vi "Data Power Output.vi"(8 "error in (no error)":errorcluster, 11 "PM-EMP in":refnum<class "PM-EMP.lvclass">) -> (0 "error out":errorcluster, 2 "Power Out":dbl, 3 "PM-EMP out":refnum<class "PM-EMP.lvclass">)   [LabVIEW 2020, in "PM-EMP.lvclass"]
uses:
  PM-EMP.lvclass
  C:/Sandbox/Git_Sandbox/WiSpry Test Framework source code (LV20)/WiSpry Test Framework/Instruments/Instrument.lvclass
  Instrument.lvclass/Instrument.ctl
  Instrument.lvclass
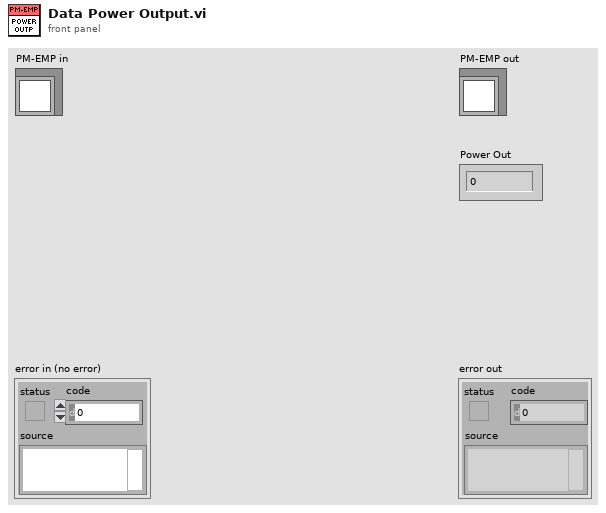
[diagram p1: front panel]
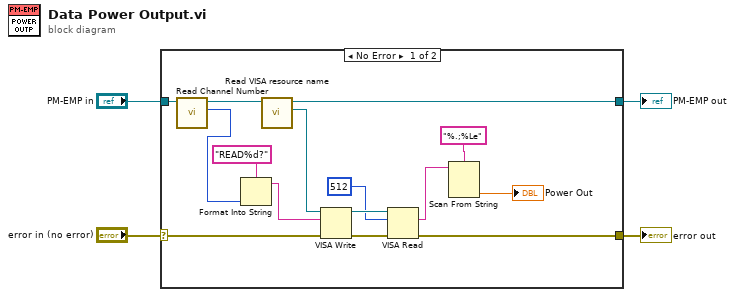
[diagram p0: block diagram]
diagram:
  n1 = case shown="No Error" "error in (no error)" {
    selector: "error in (no error)" -> [w19 w20]
    tunnel: [w9 w20] -> w3
    tunnel: "PM-EMP in" -> [w7 w21]
    tunnel: [w17 w21] -> w1
    frame No Error {
      n2 = call-dynamic "Read Channel Number.vi"("Power Meter in"=w7) -> ("Channel Number"=w5:u8, "Power Meter out"=w6:refnum<class "PM-EMP.lvclass">)  [unwired: 9 in]
      n3 = Format Into String(format string="READ%d?", w5) -> (resulting string=w14:string)  [unwired: 2 in, 1 out]
      n4 = call "Read VISA resource name.vi"("Instrument in"=w6) -> ("VISA resource name"=w18:refnum<visa-resource-name>, "Instrument out"=w17:refnum<class "PM-EMP.lvclass">)  [unwired: 9 in]
      n5 = VISA Write(VISA resource name=w18, write buffer=w14, error in (no error)=w19) -> (VISA resource name out=w13:refnum<visa-resource-name>, error out=w12:errorcluster)  [unwired: 1 out]
      n6 = VISA Read(VISA resource name=w13, byte count=u32 512, error in (no error)=w12) -> (read buffer=w10:string, error out=w9:errorcluster)  [unwired: 2 out]
      n7 = Scan From String(format string="%.;%Le", input string=w10) -> (output 1=→"Power Out":dbl)  [unwired: 3 in, 3 out]
    }
    frame Error {
    }
  }
  "error out" <- w3
  "PM-EMP out" <- w1
